vi "Connect_EventRefOut_Bool.vi"(8 "Error In":errorcluster, 10 "Signal":string, 11 "Sender In":refnum<class "LQObject.lvclass">) -> (0 "Error Out":errorcluster, 2 "Bool Signal":refnum<user-event>, 3 "Sender Out":refnum<class "LQObject.lvclass">)   [LabVIEW 2013, in "Template.lvlib" / "LQCoreEngine.lvclass"]
uses:
  LQCoreEngine.lvclass
  LQObject/LQObject.lvclass
  LQIdentity/LQIdentity.lvclass/LQIdentity.ctl
  _Private/Signals and Slots/Connection Action.ctl
  Template.lvlib
  LQIdentity/LQIdentity.lvclass
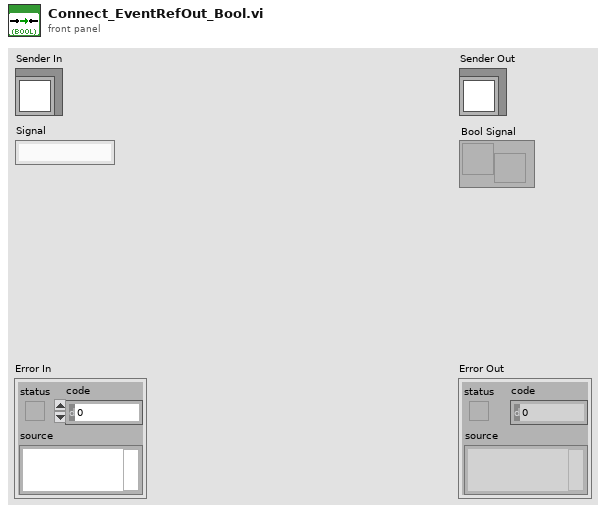
[diagram p1: front panel]
types:
  T1 = typedef "Template.lvlib/LQCoreEngine.lvclass/Connection Action.ctl" = enum16{"Init", "Add Connection", "Get Connections", "Clean Up"}
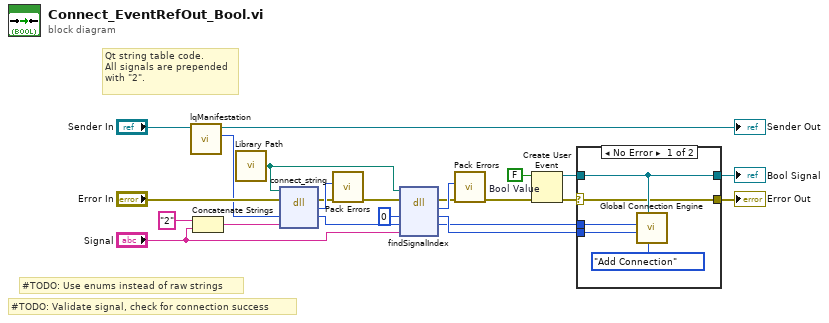
[diagram p0: block diagram]
diagram:
  w3 = FALSE  # Bool Value
  # "#TODO: Validate signal, check for connection success"
  # "Qt string table code.\nAll signals are prepended\nwith \"2\"."
  # "#TODO: Use enums instead of raw strings"
  n1 = call "lqManifestation.vi"("LQIdentity in"="Sender In") -> ("Manifestation"=w19:u64, "LQIdentity out"=→"Sender Out":refnum<class "LQObject.lvclass">)  [unwired: 9 in]
  n2 = Concatenate Strings("2" ("string"), "Signal") -> (w16:string)
  n3 = call "Library Path.vi"() -> ("Library Path"=w6:path)
  n4 = dll-call lib="?" fn="connect_string"(path in=w6, error in="Error In", "_instance"=w19, "encodedSignal"=w16) -> (error out=w11:errorcluster, "errorCode"=w12:i32, "_instance"=w18:u64)  [unwired: 2 in, 1 out]
  n5 = call "Pack Errors.vi"("Error In"=w11, "Error Code"=w12) -> ("Error Out"=w10:errorcluster)  [unwired: 9 in]
  n6 = dll-call lib="?" fn="findSignalIndex"(path in=w6, error in=w10, "retVal"=i64 0, "_instance"=w18, "encodedSignal"="Signal") -> (error out=w8:errorcluster, "errorCode"=w9:i32, "retVal"=w14:i64, "_instance"=w13:u64)  [unwired: 2 in, 1 out]
  n7 = call "Pack Errors.vi"("Error In"=w8, "Error Code"=w9) -> ("Error Out"=w7:errorcluster)  [unwired: 9 in]
  n8 = Create User Event(user event datatype=w3, error in=w7) -> (user event=w2:refnum<user-event>, error out=w5:errorcluster)
  n9 = case shown="No Error" w5 {
    selector: w5 -> [w24 w29]
    tunnel: w2 -> [w25 w30]
    tunnel: w14 -> [w28 _]
    tunnel: w13 -> [w27 _]
    tunnel: [w25 w30] -> w1
    tunnel: [w24 w29] -> w4
    frame No Error {
      n10 = call "Global Connection Engine.vi"("Connection Action"=Connection_Action."Add Connection", "Signal Channel"=w25, "Signal Index"=w28, "QObject Refnum"=w27) -> ()  [unwired: 7 in, 1 out]
    }
    frame Error {
    }
  }
  "Error Out" <- w4
  "Bool Signal" <- w1
